vi "ATSpectrograph_acceptCommand_disable.vi"(8 "error in (no error)":errorcluster, 11 "command_disable_Ctl":T1) -> (0 "error out":errorcluster, 2 "function return":i32, 3 "command_disable_Ctl out":T1)   [LabVIEW 2016, in "SALLV_ATSpectrograph.lvlib"]
doc: "int ATSpectrograph_shm_acceptCommand_disableLV(ATSpectrograph_command_disableLV *command_disable_Ctl );"
uses:
  SALLV_ATSpectrograph.lvlib
  DataTypes/command_disable.ctl
  SALLV_ATSpectrograph.so
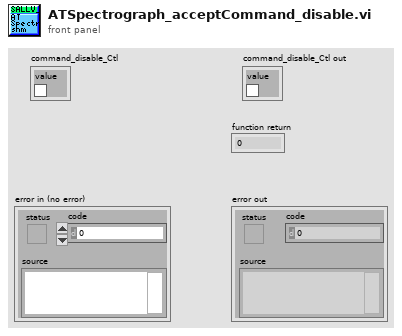
[diagram p1: front panel]
types:
  T1 = typedef "SALLV_ATSpectrograph.lvlib/command_disable.ctl" = cluster{"value":bool}
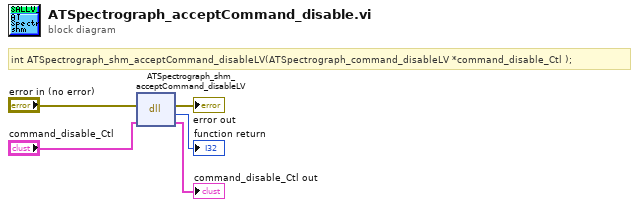
[diagram p0: block diagram]
diagram:
  # "int ATSpectrograph_shm_acceptCommand_disableLV(ATSpectrograph_command_disableLV *command_disable_Ctl );"
  n1 = dll-call lib="home/harini/tcs/SALLV_ATSpectrograph/SALLV_ATSpectrograph.*" fn="ATSpectrograph_shm_acceptCommand_disableLV"(error in="error in (no error)", "command_disable_Ctl"="command_disable_Ctl") -> (error out=→"error out":errorcluster, →"function return":i32, "command_disable_Ctl"=→"command_disable_Ctl out":T1)  [unwired: 2 in, 1 out]
